vi "Set State Button States.vi"(8 "Active":refnum<vi>, 9 "Standby":refnum<vi>, 10 "Disable":refnum<vi>, 11 "State":T1) -> ()   [LabVIEW 2015]
uses:
  System State.ctl
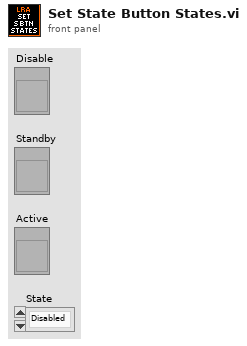
[diagram p1: front panel]
types:
  T1 = typedef "System State.ctl" = enum16{"Disabled", "E-Stop", "Standby", "Active"}
  T2 = enum8{"Enabled", "Disabled", "Disabled and Grayed Out"}
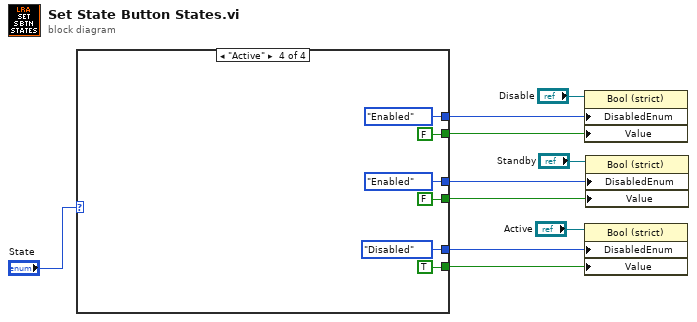
[diagram p0: block diagram]
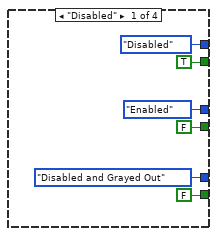
[diagram p2: hidden frame]
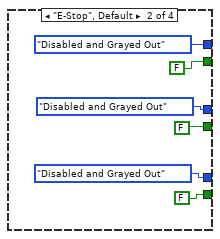
[diagram p3: hidden frame]
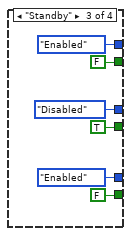
[diagram p4: hidden frame]
diagram:
  n1 = case shown="\"Active\"" "State" {
    tunnel: [T2."Disabled" ("Disabled") T2."Disabled and Grayed Out" ("Disabled") T2."Enabled" ("Disabled") T2."Enabled" ("Disabled")] -> w6
    tunnel: [T2."Enabled" ("Disabled") T2."Disabled and Grayed Out" ("Disabled") T2."Disabled" ("Disabled") T2."Enabled" ("Disabled")] -> w5
    tunnel: [T2."Disabled and Grayed Out" ("Disabled") T2."Disabled and Grayed Out" ("Disabled") T2."Enabled" ("Disabled") T2."Disabled" ("Disabled")] -> w4
    tunnel: [TRUE FALSE FALSE FALSE] -> w3
    tunnel: [FALSE FALSE TRUE FALSE] -> w2
    tunnel: [FALSE FALSE FALSE TRUE] -> w1
    frame "Disabled" {
    }
    frame "E-Stop", Default {
    }
    frame "Standby" {
    }
    frame "Active" {
    }
  }
  n2 = property class="Bool (strict)"(reference="Disable", "DisabledEnum"=w6, "Value"=w3) -> ()  [unwired: 1 in, 2 out]
  n3 = property class="Bool (strict)"(reference="Active", "DisabledEnum"=w4, "Value"=w1) -> ()  [unwired: 1 in, 2 out]
  n4 = property class="Bool (strict)"(reference="Standby", "DisabledEnum"=w5, "Value"=w2) -> ()  [unwired: 1 in, 2 out]
